vi "菜单练习.vi"() -> ()   [LabVIEW 2018]
panel:
  in  "机种名称":string
  out "Row":i32
  in  "机种文件":i32(listbox)
  in  "停止":bool
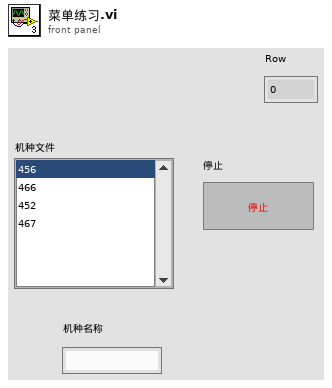
[diagram p1: front panel]
types:
  T1 = typedef "LVPoint32TypeDef.ctl" = cluster{"Horizontal":i32, "Vertical":i32}
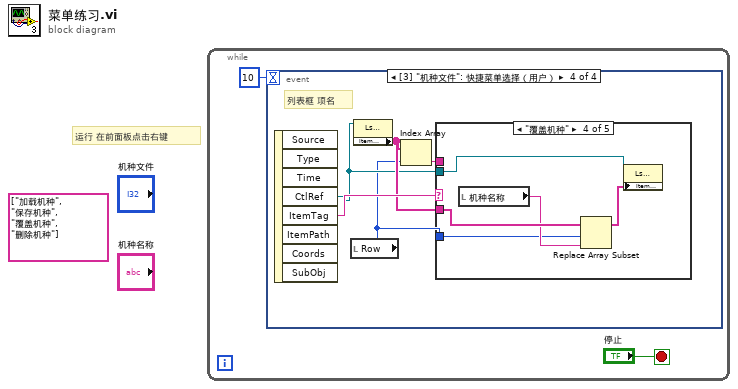
[diagram p0: block diagram]
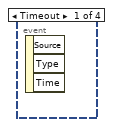
[diagram p2: hidden frame]
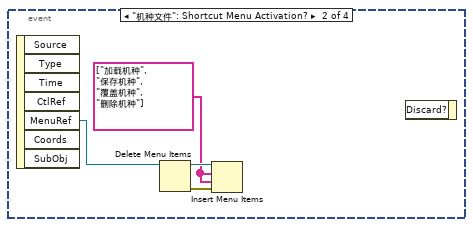
[diagram p3: hidden frame]
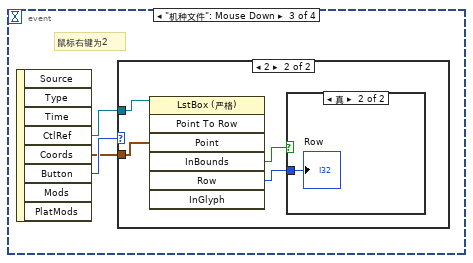
[diagram p4: hidden frame]
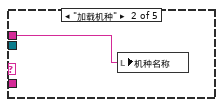
[diagram p8: hidden frame]
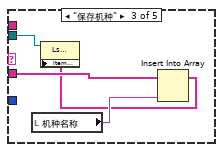
[diagram p9: hidden frame]
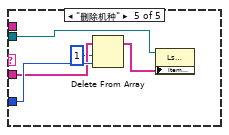
[diagram p10: hidden frame]
diagram:
  (unwired) string[] ["加载机种", "保存机种", "覆盖机种", "删除机种"] ("项标识符")
  # "运行 在前面板点击右键"
  n1 = while {
    stop <- "停止" stop-if-true
    n2 = event shown="[3] \"机种文件\": 快捷菜单选择（用户）" {
      selector: _ -> [_ _ _ _]
      dyn-events: _ -> [_ _ _ _]
      timeout: 10 -> [_ _ _ _]
      event Timeout {
        n3 = event-data() -> ()  [unwired: 1 in, 3 out]
      }
      event "机种文件": Shortcut Menu Activation? {
        w4 = string[] ["加载机种", "保存机种", "覆盖机种", "删除机种"] ("项标识符")
        n4 = event-data() -> ("MenuRef"=w3:refnum<k9>)  [unwired: 1 in, 6 out]
        n5 = Delete Menu Items(9:w3) -> (0:w6:errorcluster, 3:w5:refnum<k9>)  [unwired: 3 in]
        n6 = Insert Menu Items(6:w6, 7:w4, 8:w4, 9:w5) -> ()  [unwired: 2 in, 3 out]
        n7 = event-data() -> ()  [unwired: 2 in, 1 out]
      }
      event "机种文件": Mouse Down {
        # "鼠标右键为2"
        n8 = event-data() -> ("CtlRef"=w8:refnum<vi>, "Coords"=w7:T1, "Button"=w9:u16)  [unwired: 1 in, 5 out]
        n9 = case shown="2" w9 {
          tunnel: w8 -> [_ w12]
          tunnel: w7 -> [_ w13]
          frame 0, Default {
          }
          frame 2 {
            n10 = invoke class="LstBox (严格)" method="Point To Row"(reference=w12, "Point"=w13) -> ("InBounds"=w11:bool, "Row"=w10:i32)  [unwired: 5 in, 5 out]
            n11 = case shown="真" w11 {
              tunnel: w10 -> [_ w14]
              frame False {
              }
              frame True {
                "Row" <- w14
              }
            }
          }
        }
      }
      event "机种文件": Shortcut Menu Selection (User) {
        # "列表框 项名"
        n12 = event-data() -> ("CtlRef"=w16:refnum<vi>, "ItemTag"=w19:string)  [unwired: 1 in, 6 out]
        n13 = local read "Row"() -> (w15:i32)
        n14 = property class="LstBox (严格)"(reference=w16) -> ("Item Names"=w17:string[])  [unwired: 1 in, 2 out]
        n15 = Index Array(array=w17, index=w15) -> (element=w18:string)
        n16 = case shown="\"覆盖机种\"" w19 {
          tunnel: w18 -> [_ w20 _ _ _]
          tunnel: w17 -> [_ _ w24 w29 w33]
          tunnel: w16 -> [_ _ w23 w26 w30]
          tunnel: w15 -> [_ _ _ w27 w34]
          frame "假", Default {
          }
          frame "加载机种" {
            n17 = local write "机种名称"(w20) -> ()
          }
          frame "保存机种" {
            n18 = local read "机种名称"() -> (w22:string)
            n19 = Insert Into Array(array=w24, new element=w22) -> (w21:string[])  [unwired: 1 in]
            n20 = property class="LstBox (严格)"(reference=w23, "Item Names"=w21) -> ()  [unwired: 1 in, 2 out]
          }
          frame "覆盖机种" {
            n21 = local read "机种名称"() -> (w28:string)
            n22 = Replace Array Subset(array=w29, new element=w28, index=w27) -> (w25:string[])
            n23 = property class="LstBox (严格)"(reference=w26, "Item Names"=w25) -> ()  [unwired: 1 in, 2 out]
          }
          frame "删除机种" {
            n24 = Delete From Array(array=w33, length=1 ("长度"), index=w34) -> (array with subset deleted=w31:string[])  [unwired: 1 out]
            n25 = property class="LstBox (严格)"(reference=w30, "Item Names"=w31) -> ()  [unwired: 1 in, 2 out]
          }
        }
      }
    }
  }
